vi "Pcre2GetMatchDataHeapframesSize.vi"(8 "error in":errorcluster, 11 "pMatchData":u64 format="%.0x") -> (0 "error out":errorcluster, 2 "HeapFramesSize":u64, 3 "pMatchData":u64 format="%.0x")   [LabVIEW 2021, in "libpcre2-8.lvlib"]
uses:
  libpcre2-8.lvlib
  libpcre2-8-x32.dll
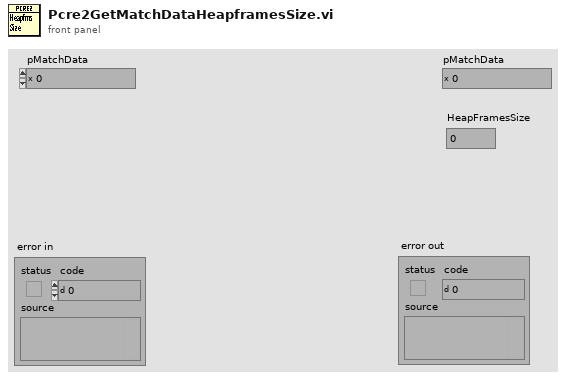
[diagram p1: front panel]
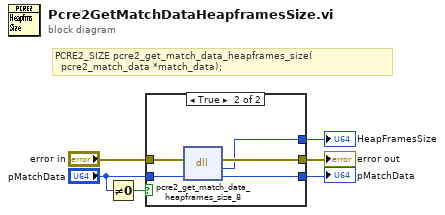
[diagram p0: block diagram]
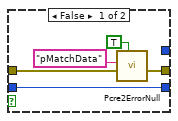
[diagram p2: hidden frame]
diagram:
  # "PCRE2_SIZE pcre2_get_match_data_heapframes_size(\n  pcre2_match_data *match_data);"
  n1 = Not Equal To 0?(x="pMatchData") -> (x != 0?=w1:bool)
  n2 = case shown="True" w1 {
    tunnel: "error in" -> [w9 w16]
    tunnel: [w10 w15] -> w5
    tunnel: [_ w14] -> w4
    tunnel: [w11 w13] -> w3
    tunnel: "pMatchData" -> [w11 w12]
    frame False {
      n3 = call "Pcre2ErrorNull.vi"("IsPointer? (F)"=TRUE, "error in"=w9, "What"="pMatchData") -> ("error out"=w10:errorcluster)  [unwired: 8 in]
    }
    frame True {
      n4 = dll-call lib="libpcre2-8-x*.dll" fn="pcre2_get_match_data_heapframes_size_8"(error in=w16, "match_data"=w12) -> (error out=w15:errorcluster, "HeapfremesSize"=w14:u64, "match_data"=w13:u64)  [unwired: 2 in, 1 out]
    }
  }
  "error out" <- w5
  "pMatchData" <- w3
  "HeapFramesSize" <- w4
